vi "add_stop_for_sync.vi"(9 "Instructions Out":T1(array[cluster])=[{"Instruct Data"=0, "Op Code"=0, "Flags"=[FALSE, FALSE, FALSE, FALSE, FALSE, TRUE, TRUE, TRUE, FALSE, FALSE, FALSE, TRUE, TRUE, FALSE, FALSE, TRUE, TRUE, FALSE, FALSE, FALSE, TRUE, FALSE, TRUE, FALSE], "Comments"="", "Time (s)"=5e-08}, {"Instruct Data"=0, "Op Code"=8, "Flags"=[FALSE, FALSE, FALSE, FALSE, FALSE, TRUE, TRUE, TRUE, FALSE, FALSE, FALSE, TRUE, TRUE, FALSE, FALSE, TRUE, TRUE, FALSE, FALSE, FALSE, TRUE, FALSE, TRUE, FALSE], "Comments"="", "Time (s)"=0.1}, {"Instruct Data"=7, "Op Code"=0, "Flags"=[TRUE, FALSE, FALSE, FALSE, TRUE, TRUE, FALSE, TRUE, FALSE, TRUE, FALSE, TRUE, FALSE, FALSE, FALSE, TRUE, TRUE, TRUE, FALSE, FALSE, TRUE, FALSE, TRUE, FALSE], "Comments"="Blue MOT", "Time (s)"=2.5}, {"Instruct Data"=9, "Op Code"=0, "Flags"=[TRUE, FALSE, FALSE, FALSE, FALSE, TRUE, FALSE, TRUE, FALSE, TRUE, FALSE, TRUE, TRUE, FALSE, FALSE, TRUE, TRUE, TRUE, FALSE, FALSE, TRUE, FALSE, TRUE, FALSE], "Comments"="Hold", "Time (s)"=0.1}, {"Instruct Data"=9, "Op Code"=0, "Flags"=[TRUE, FALSE, FALSE, FALSE, FALSE, FALSE, FALSE, TRUE, FALSE, TRUE, FALSE, TRUE, TRUE, FALSE, FALSE, TRUE, TRUE, FALSE, FALSE, FALSE, TRUE, FALSE, TRUE, FALSE], "Comments"="Repump", "Time (s)"=0.05}, {"Instruct Data"=9, "Op Code"=0, "Flags"=[FALSE, FALSE, FALSE, FALSE, FALSE, TRUE, TRUE, FALSE, TRUE, FALSE, FALSE, TRUE, TRUE, FALSE, FALSE, TRUE, TRUE, FALSE, FALSE, FALSE, TRUE, FALSE, TRUE, FALSE], "Comments"="Red MOT", "Time (s)"=0.2}, {"Instruct Data"=10, "Op Code"=0, "Flags"=[FALSE, FALSE, FALSE, FALSE, FALSE, TRUE, TRUE, FALSE, TRUE, FALSE, FALSE, TRUE, TRUE, FALSE, FALSE, TRUE, FALSE, FALSE, FALSE, FALSE, FALSE, FALSE, TRUE, FALSE], "Comments"="Load ODT", "Time (s)"=0.1}, {"Instruct Data"=5, "Op Code"=2, "Flags"=[FALSE, FALSE, FALSE, FALSE, FALSE, TRUE, TRUE, TRUE, FALSE, FALSE, FALSE, TRUE, TRUE, FALSE, FALSE, TRUE, FALSE, FALSE, FALSE, FALSE, FALSE, TRUE, TRUE, FALSE], "Comments"="ODT Hold", "Time (s)"=0.5}, {"Instruct Data"=7, "Op Code"=3, "Flags"=[FALSE, FALSE, FALSE, FALSE, FALSE, TRUE, TRUE, TRUE, FALSE, FALSE, FALSE, TRUE, TRUE, FALSE, FALSE, TRUE, FALSE, FALSE, FALSE, FALSE, FALSE, TRUE, TRUE, FALSE], "Comments"="hold for mcs", "Time (s)"=0.05}, {"Instruct Data"=0, "Op Code"=0, "Flags"=[FALSE, FALSE, FALSE, FALSE, FALSE, TRUE, TRUE, TRUE, FALSE, FALSE, FALSE, TRUE, TRUE, FALSE, FALSE, TRUE, TRUE, FALSE, FALSE, FALSE, TRUE, FALSE, TRUE, FALSE], "Comments"="Drop", "Time (s)"=0.01}, {"Instruct Data"=0, "Op Code"=0, "Flags"=[FALSE, TRUE, TRUE, TRUE, FALSE, TRUE, TRUE, TRUE, FALSE, FALSE, FALSE, TRUE, TRUE, FALSE, FALSE, TRUE, TRUE, FALSE, FALSE, FALSE, TRUE, FALSE, TRUE, FALSE], "Comments"="Image atoms ", "Time (s)"=1e-05}, {"Instruct Data"=0, "Op Code"=0, "Flags"=[FALSE, FALSE, FALSE, FALSE, FALSE, TRUE, TRUE, TRUE, FALSE, FALSE, FALSE, TRUE, TRUE, FALSE, FALSE, TRUE, TRUE, FALSE, FALSE, FALSE, TRUE, FALSE, TRUE, FALSE], "Comments"="Wait", "Time (s)"=0.081}, {"Instruct Data"=0, "Op Code"=0, "Flags"=[FALSE, TRUE, TRUE, TRUE, FALSE, TRUE, TRUE, TRUE, FALSE, FALSE, FALSE, TRUE, TRUE, FALSE, FALSE, TRUE, TRUE, FALSE, FALSE, FALSE, TRUE, FALSE, TRUE, FALSE], "Comments"="Image BG", "Time (s)"=1e-05}, {"Instruct Data"=0, "Op Code"=6, "Flags"=[FALSE, FALSE, FALSE, FALSE, FALSE, TRUE, TRUE, TRUE, FALSE, FALSE, FALSE, TRUE, TRUE, FALSE, FALSE, TRUE, TRUE, FALSE, FALSE, FALSE, TRUE, FALSE, TRUE, FALSE], "Comments"="Kill time", "Time (s)"=0.15}] caption="Instructions" {"Time (s)" min=5e-08 format="%.3p"; "Op Code" items=["Continue", "Stop", "Loop", "End Loop", "JSR", "RTS", "Branch", "Long Delay", "Wait"]; "Instruct Data" format="%#.2p"}) -> (1 "Instructions Out 2":T1(array[cluster])=[{"Instruct Data"=0, "Op Code"=0, "Flags"=[FALSE, FALSE, FALSE, FALSE, FALSE, TRUE, TRUE, TRUE, FALSE, FALSE, FALSE, TRUE, TRUE, FALSE, FALSE, TRUE, TRUE, FALSE, FALSE, FALSE, TRUE, FALSE, TRUE, FALSE], "Comments"="", "Time (s)"=5e-08}, {"Instruct Data"=0, "Op Code"=8, "Flags"=[FALSE, FALSE, FALSE, FALSE, FALSE, TRUE, TRUE, TRUE, FALSE, FALSE, FALSE, TRUE, TRUE, FALSE, FALSE, TRUE, TRUE, FALSE, FALSE, FALSE, TRUE, FALSE, TRUE, FALSE], "Comments"="", "Time (s)"=0.1}, {"Instruct Data"=7, "Op Code"=0, "Flags"=[TRUE, FALSE, FALSE, FALSE, TRUE, TRUE, FALSE, TRUE, FALSE, TRUE, FALSE, TRUE, FALSE, FALSE, FALSE, TRUE, TRUE, TRUE, FALSE, FALSE, TRUE, FALSE, TRUE, FALSE], "Comments"="Blue MOT", "Time (s)"=2.5}, {"Instruct Data"=9, "Op Code"=0, "Flags"=[TRUE, FALSE, FALSE, FALSE, FALSE, TRUE, FALSE, TRUE, FALSE, TRUE, FALSE, TRUE, TRUE, FALSE, FALSE, TRUE, TRUE, TRUE, FALSE, FALSE, TRUE, FALSE, TRUE, FALSE], "Comments"="Hold", "Time (s)"=0.1}, {"Instruct Data"=9, "Op Code"=0, "Flags"=[TRUE, FALSE, FALSE, FALSE, FALSE, FALSE, FALSE, TRUE, FALSE, TRUE, FALSE, TRUE, TRUE, FALSE, FALSE, TRUE, TRUE, FALSE, FALSE, FALSE, TRUE, FALSE, TRUE, FALSE], "Comments"="Repump", "Time (s)"=0.05}, {"Instruct Data"=9, "Op Code"=0, "Flags"=[FALSE, FALSE, FALSE, FALSE, FALSE, TRUE, TRUE, FALSE, TRUE, FALSE, FALSE, TRUE, TRUE, FALSE, FALSE, TRUE, TRUE, FALSE, FALSE, FALSE, TRUE, FALSE, TRUE, FALSE], "Comments"="Red MOT", "Time (s)"=0.2}, {"Instruct Data"=10, "Op Code"=0, "Flags"=[FALSE, FALSE, FALSE, FALSE, FALSE, TRUE, TRUE, FALSE, TRUE, FALSE, FALSE, TRUE, TRUE, FALSE, FALSE, TRUE, FALSE, FALSE, FALSE, FALSE, FALSE, FALSE, TRUE, FALSE], "Comments"="Load ODT", "Time (s)"=0.1}, {"Instruct Data"=5, "Op Code"=2, "Flags"=[FALSE, FALSE, FALSE, FALSE, FALSE, TRUE, TRUE, TRUE, FALSE, FALSE, FALSE, TRUE, TRUE, FALSE, FALSE, TRUE, FALSE, FALSE, FALSE, FALSE, FALSE, TRUE, TRUE, FALSE], "Comments"="ODT Hold", "Time (s)"=0.5}, {"Instruct Data"=7, "Op Code"=3, "Flags"=[FALSE, FALSE, FALSE, FALSE, FALSE, TRUE, TRUE, TRUE, FALSE, FALSE, FALSE, TRUE, TRUE, FALSE, FALSE, TRUE, FALSE, FALSE, FALSE, FALSE, FALSE, TRUE, TRUE, FALSE], "Comments"="hold for mcs", "Time (s)"=0.05}, {"Instruct Data"=0, "Op Code"=0, "Flags"=[FALSE, FALSE, FALSE, FALSE, FALSE, TRUE, TRUE, TRUE, FALSE, FALSE, FALSE, TRUE, TRUE, FALSE, FALSE, TRUE, TRUE, FALSE, FALSE, FALSE, TRUE, FALSE, TRUE, FALSE], "Comments"="Drop", "Time (s)"=0.01}, {"Instruct Data"=0, "Op Code"=0, "Flags"=[FALSE, TRUE, TRUE, TRUE, FALSE, TRUE, TRUE, TRUE, FALSE, FALSE, FALSE, TRUE, TRUE, FALSE, FALSE, TRUE, TRUE, FALSE, FALSE, FALSE, TRUE, FALSE, TRUE, FALSE], "Comments"="Image atoms ", "Time (s)"=1e-05}, {"Instruct Data"=0, "Op Code"=0, "Flags"=[FALSE, FALSE, FALSE, FALSE, FALSE, TRUE, TRUE, TRUE, FALSE, FALSE, FALSE, TRUE, TRUE, FALSE, FALSE, TRUE, TRUE, FALSE, FALSE, FALSE, TRUE, FALSE, TRUE, FALSE], "Comments"="Wait", "Time (s)"=0.081}, {"Instruct Data"=0, "Op Code"=0, "Flags"=[FALSE, TRUE, TRUE, TRUE, FALSE, TRUE, TRUE, TRUE, FALSE, FALSE, FALSE, TRUE, TRUE, FALSE, FALSE, TRUE, TRUE, FALSE, FALSE, FALSE, TRUE, FALSE, TRUE, FALSE], "Comments"="Image BG", "Time (s)"=1e-05}, {"Instruct Data"=0, "Op Code"=6, "Flags"=[FALSE, FALSE, FALSE, FALSE, FALSE, TRUE, TRUE, TRUE, FALSE, FALSE, FALSE, TRUE, TRUE, FALSE, FALSE, TRUE, TRUE, FALSE, FALSE, FALSE, TRUE, FALSE, TRUE, FALSE], "Comments"="Kill time", "Time (s)"=0.15}] caption="Instructions" {"Time (s)" min=5e-08 format="%.3p"; "Op Code" items=["Continue", "Stop", "Loop", "End Loop", "JSR", "RTS", "Branch", "Long Delay", "Wait"]; "Instruct Data" format="%#.2p"})   [LabVIEW 2015]
panel:
  # "1"
  # "2"
  # "3"
  # "4"
  # "5"
  # "6"
  # "7"
  # "8"
  # "9"
  # "10"
  # "11"
  # "12"
  # "13"
  # "14"
  # "15"
  # "16"
  # "17"
  # "18"
  # "19"
  # "20"
  # "21"
  # "22"
  # "23"
  # "24"
  # "1"
  # "2"
  # "3"
  # "4"
  # "5"
  # "6"
  # "7"
  # "8"
  # "9"
  # "10"
  # "11"
  # "12"
  # "13"
  # "14"
  # "15"
  # "16"
  # "17"
  # "18"
  # "19"
  # "20"
  # "21"
  # "22"
  # "23"
  # "24"
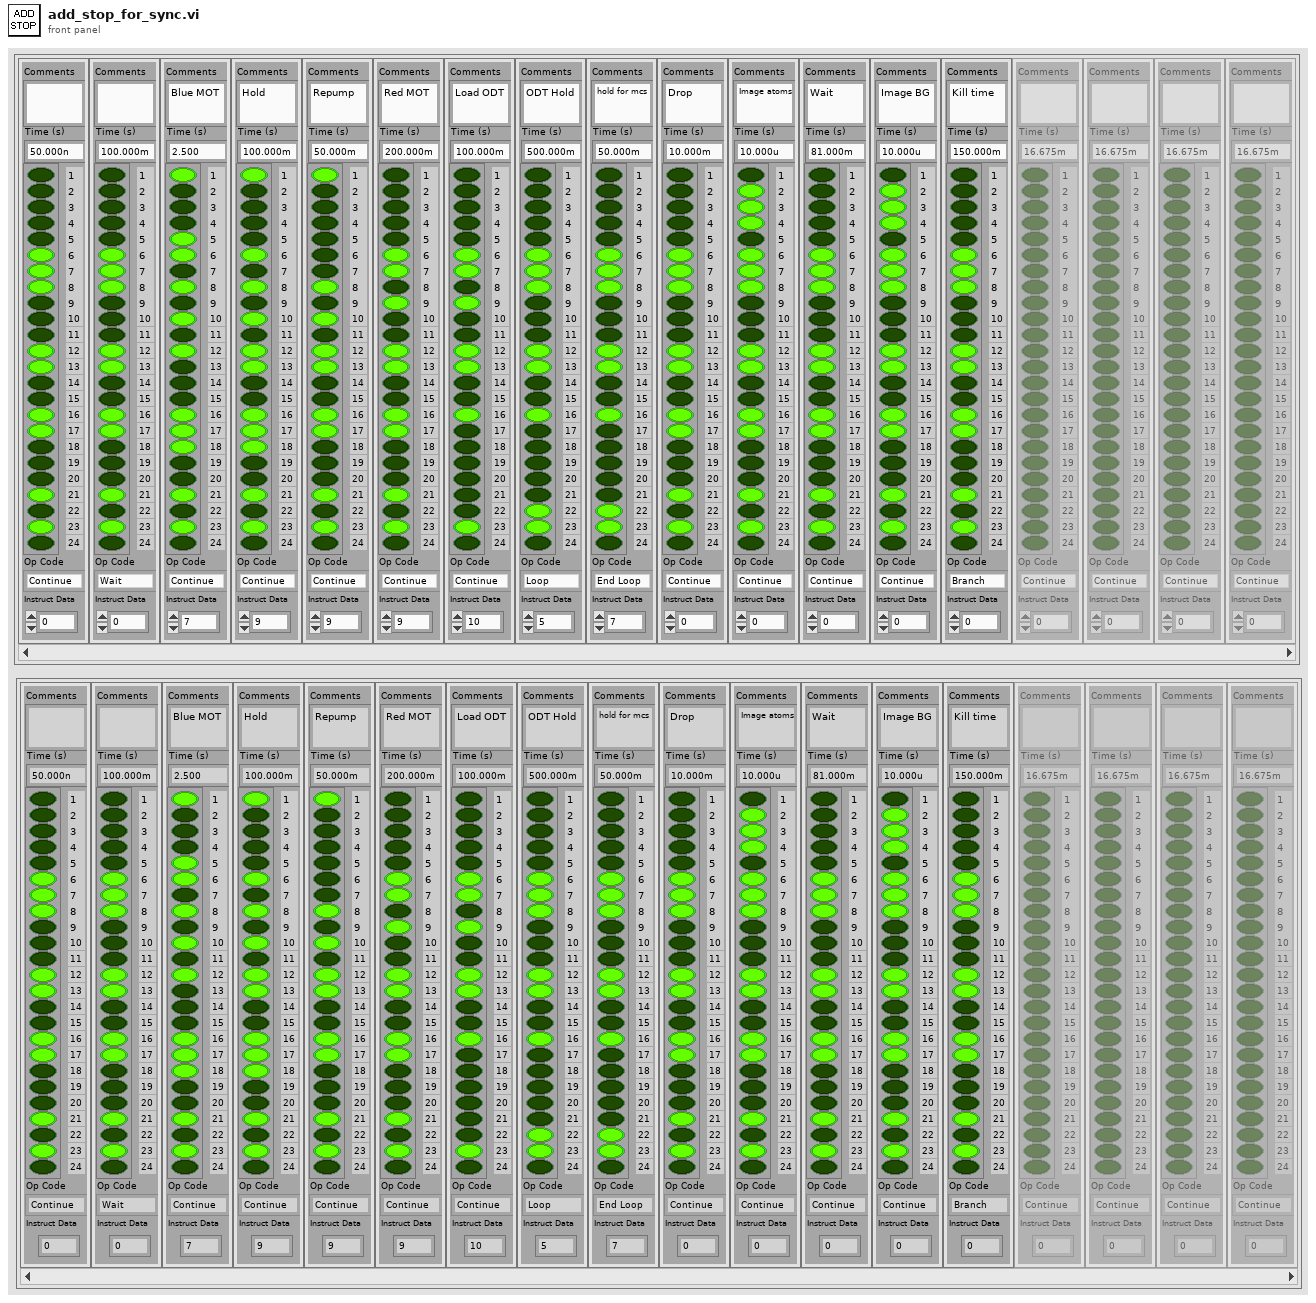
[diagram p1: front panel]
types:
  T1 = cluster{"Instruct Data":i32, "Op Code":i32, "Flags":bool[], "Comments":string, "Time (s)":dbl}[]
  T2 = cluster{"Instruct Data":i32, "Op Code":i32, "Flags":bool[], "Comments":string, "Time (s)":dbl}
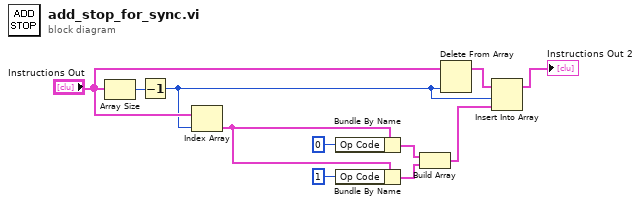
[diagram p0: block diagram]
diagram:
  n1 = Array Size(array="Instructions Out") -> (size(s)=w11:i32)
  n2 = Decrement(x=w11) -> (x-1=w4:i32)
  n3 = Index Array(array="Instructions Out", index=w4) -> (element=w10:T2)
  n4 = Bundle By Name(cluster=w10, "Op Code"=0) -> (w7:T2)
  n5 = Bundle By Name(cluster=w10, "Op Code"=1) -> (w6:T2)
  n6 = Build Array(w7, w6) -> (w2:T1)
  n7 = Delete From Array(array="Instructions Out", index=w4) -> (array with subset deleted=w3:T1)  [unwired: 1 in, 1 out]
  n8 = Insert Into Array(array=w3, index=w4, new element=w2) -> (→"Instructions Out 2":T1)
